vi "nn_train.vi"() -> ()   [LabVIEW 2023]
panel:
  out "Y out":dbl[](array[numeric])
  out "Array":i32[](array[numeric])
  in  "learning rate":dbl
  in  "number of iterations":i32
  in  "Path":path
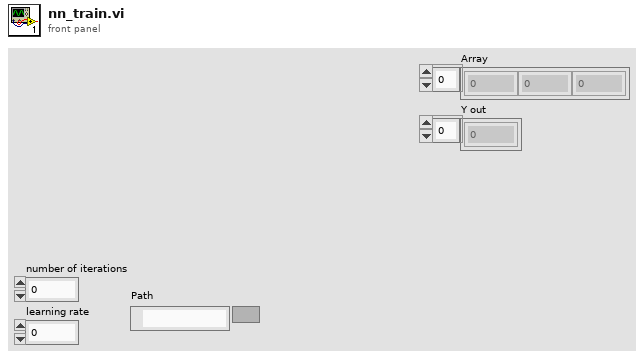
[diagram p1: front panel]
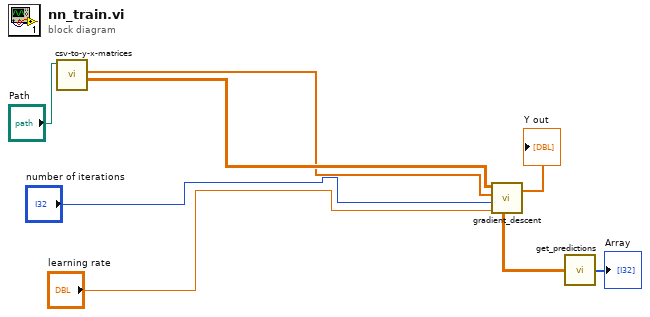
[diagram p0: block diagram]
diagram:
  n1 = call "csv-to-y-x-matrices.vi"("Path"="Path") -> ("X"=w7:dbl[][], "Y"=w6:dbl[])  [unwired: 7 in, 2 out]
  n2 = call "gradient_descent.vi"("alpha"="learning rate", "iterations"="number of iterations", "Y in"=w6, "X in"=w7) -> ("predictions"=w3:dbl[][], "Y out"=→"Y out":dbl[])  [unwired: 6 out]
  n3 = call "get_predictions.vi"("2D array"=w3) -> ("Array"=→"Array":i32[])
